vi "compress.vi"   [LabVIEW 2015, in "lv-bin-7zip.lvlib" / "v1.lvlib"]
uses:
  v1.lvlib
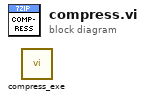
[diagram p0: block diagram]
diagram:
  n1 = call "compress_exe.vi"() -> ()  [unwired: 10 in, 2 out]
